vi "Save bline to memory1.vi"(0 "PSOCTSpectral Bline":u16[](array[numeric]), 1 "action":T1=enum."Save(ThorOCT)", 5 "index (row)":i32, 9 "PSOCT Spatial Bline":sgl[](array[numeric]), 11 "error in":errorcluster) -> (15 "error out":errorcluster)   [LabVIEW 2018]
uses:
  Controls/Save Bline to Mem Control.ctl
  Controls/FGV Actions.ctl
  Controls/Queue Manager Actions.ctl
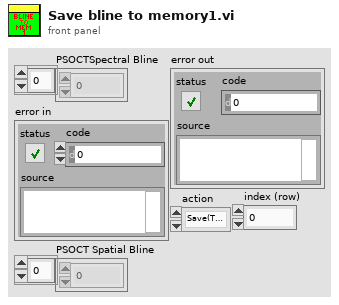
[diagram p1: front panel]
types:
  T1 = typedef "Save Bline to Mem Control.ctl" = enum16{"Output data", "Save(ThorOCT)", "Save(PSOCT)", "FFT and Save", "Uninit", "PSOCT Spectral buffer Set", "PSOCT Spatial buffer Set", "PSOCT Spectral buffer Init", "PSOCT Spatial buffer Init", "ThorOCT Spectral buffer Init", "ThorOCT Spatial buffer Init", "ThorOCT Spectral buffer Set", "ThorOCT Spatial buffer Set", "ThorOCT Spectral Save", "Alazar Spectral Save", "PSOCT save all", "Average"}
  T2 = typedef "FGV Actions.ctl" = enum16{"Init", "Set", "Get", "Clear"}
  T3 = typedef "System Parameters.ctl" = cluster{"Optical Parameters":T4, "Vibratome":T5, "Table Stages":T6, "Imaging Parameter":T9, "Galvo HW Parameters":cluster{"Analog Out Channel":tag, "Min Voltage":dbl, "Max Voltage":dbl, "Pixel Clock Source":tag, "Sample Rate":dbl, "Line Clock Out Ch":tag, "2P ready check":tag}, "Alazar parameters":T11, "Mosaic Paramter":T18, "Manual Controls":T19, "Z stage setting":T23, "Attenuator":T24}
  T4 = typedef "Optical Parameters.ctl" = cluster{"Obj. Focal Length [mm]":dbl, "Scan Lens EFL[mm]":dbl, "Tube Lens EFL[mm]":dbl, "Galvo V Range (+/-)":dbl, "Galvo Max Half Angle [Deg]":dbl, "Max Galvo Range[%]":dbl}
  T5 = typedef "Vibratome Parameters.ctl" = cluster{"Pre Cut Dwell [s]":dbl, "Blade Frequency [RPM]":u16, "Slice Speed [mm/s]":dbl, "Post Cut Dwell [s]":dbl, "Ramp Time [s]":dbl, "Start X [mm]":dbl, "Start Y [mm]":dbl, "Slice Length [mm]":dbl, "Slice Axis":enum16{"X Axis", "Y Axis", "Z Axis"}, "Controller VISA Ref":refnum<visa-resource-name>}
  T6 = typedef "Translation Stage Parameters.ctl" = cluster{"X Stage":T7, "Y Stage":T7, "Z Stage":T7, "Attenuator":T7}
  T7 = typedef "Translation Stage Cluster.ctl" = cluster{"Position":dbl, "Is.Enabled?":bool, "Is.Connected?":bool, "Device SN":string, "AccelerationMaximum":dbl, "VelocityMaximum":dbl, "Acceleration":dbl, "Velocity":dbl, "waitTimeout (ms)":i32, "Model":T8, "Is.Homed?":bool, "MOVE":bool}
  T8 = typedef "Translation Stage Types.ctl" = enum16{"None", "Thorlabs LTS", "Thorlabs MLJ"}
  T9 = typedef "Imaging Parameters.ctl" = cluster{"Raster Scan Direction":T10, "Pixel Dwell Time [Clock Cycles]":u16, "Flyback Time [Clock Cycles]":u16, "XY Center [um]":cluster{"X":dbl, "Y":dbl}, "Pixel Step Size [um] X":dbl, "XY Image Size":enum16{"32 x 32", "64 x 64", "128 x 128", "256 x 256", "512 x 512", "1024 x 1024", "2048 x 2048"}, "Custom":bool, "Custom Size":cluster{"X":u16, "Y":u16}, "Line Averages":u16, "Pixel Step Size [um] Y":dbl}
  T10 = typedef "Scan Direction.ctl" = enum16{"Uni Directional", "Bi Directional", "None"}
  T11 = typedef "Alazar parameters.ctl" = cluster{"Trigger Settings":cluster{"General Trigger Settings":T12, "Trigger Engine 1":T13, "Trigger Engine 2":T13}, "Device ID":T14, "Ch A Input Control":T15, "Ch B Input Control":T15, "Acq Settings":T16, "Capture Clock":T17}
  T12 = typedef "General Trigger Settings.ctl" = cluster{"Trigger Operation":u32, "Coupling ID":u32, "Range ID":u32, "Delay":u32, "Timeout Ticks":u32, "Mode":u32, "Parameter":u32}
  T13 = typedef "Trigger Engine Controls.ctl" = cluster{"Trigger Engine":u32, "Source":u32, "Slope":u32, "Level":u32}
  T14 = typedef "Alazar Device ID.ctl" = cluster{"System ID":u32, "Board ID":u32}
  T15 = typedef "Channel Input Controls.ctl" = cluster{"Channel":u8, "Coupling":u32, "Range":u32, "Impedance":u32}
  T16 = typedef "Alazar Acquisition Settings.ctl" = cluster{"Record Length":u32, "Offset":u32, "Records Per Buffer":u32, "Records Count (Records/Acq)":u32, "Window Type":u32, "Footer":u32, "Samples per record":u32, "Output Format":u32}
  T17 = typedef "Clock Controls.ctl" = cluster{"Sample Rate":u32, "Decimation":u32, "Source":u32, "Edge":u32}
  T18 = typedef "Mosaic Parameter.ctl" = cluster{"X Axis":cluster{"Start [mm]":dbl, "Steps [pts]":dbl, "End [mm]":dbl}, "Y Axis":cluster{"Start [mm]":dbl, "Steps [pts]":dbl, "End [mm]":dbl}, "Scan Pattern":enum16{"Uni-directional", "Bi-Directional", "Spiral Out", "Spiral In"}, "Overlap Options":cluster{"Overlap Type":enum16{"No Overlap", "X Only", "Y Only", "X and Y"}, "Percent Overlap":u8, "Justify":enum16{"Start", "Center", "End"}}}
  T19 = typedef "Manual Controls.ctl" = cluster{"Data Path":path, "Save parameters":T20, "Acquisition mode":T21, "PSOCT Channel":u32, "Save data?":bool, "AIP rotation angle":dbl, "Pause acquisition?":bool, "Outgoing Mail Server (SMTP)":string, "Email":string, "Password":string, "Carrier 1":enum16{"T-Mobile", "AT&T", "Verizon", "Sprint"}, "phone number 1":string, "Subject":string, "Message":string, "Carrier 2":enum16{"T-Mobile", "AT&T", "Verizon", "Sprint"}, "phone number 2":string, "Outputs for GPU FFT":T22, "Slice# init":i32}
  T20 = typedef "FFT parameters.ctl" = cluster{"start pixel":i32, "#pixels to save":i32}
  T21 = typedef "FFT mode.ctl" = enum16{"ThorOCT B line", "ThorOCT Spectral", "ThorOCT FFT", "Alazar B line", "Alazar FFT", "GPU FFT", "Alazar Spectral", "Simulation", "auto adjust focus", "Save all"}
  T22 = typedef "GPU FFT outputs.ctl" = enum16{"Amp + Phase diff", "Amp + Phase", "Amp only"}
  T23 = typedef "Vibratome Param.ctl" = cluster{"first cut height(mm)":dbl, "cut thickness[um]":u32[], "#cycles":u16, "PSOCT thickness(um)":u32[], "First image height(mm)":dbl, "Pause?":bool[], "Z0":dbl, "fixed Z0?":bool, "Cut_aft_2P?(leave empty if no 2P)":bool[], "2P thickness(um) (leave empty if not used)":u32[], "2P_cover_all_depth? (leave empty if no 2P)":bool[]}
  T24 = typedef "attenuator.ctl" = cluster{"Power after Objective (recalibrate every 6 month)":dbl[]}
  T25 = typedef "Queue Manager Actions.ctl" = enum16{"Init", "Enqueue", "Enqueue All", "Preview Queue", "Dequeue", "Get Status", "Flush Queue", "Flush All Queues", "Release All Queues", "Release Queue", "Enqueue at Opposite End"}
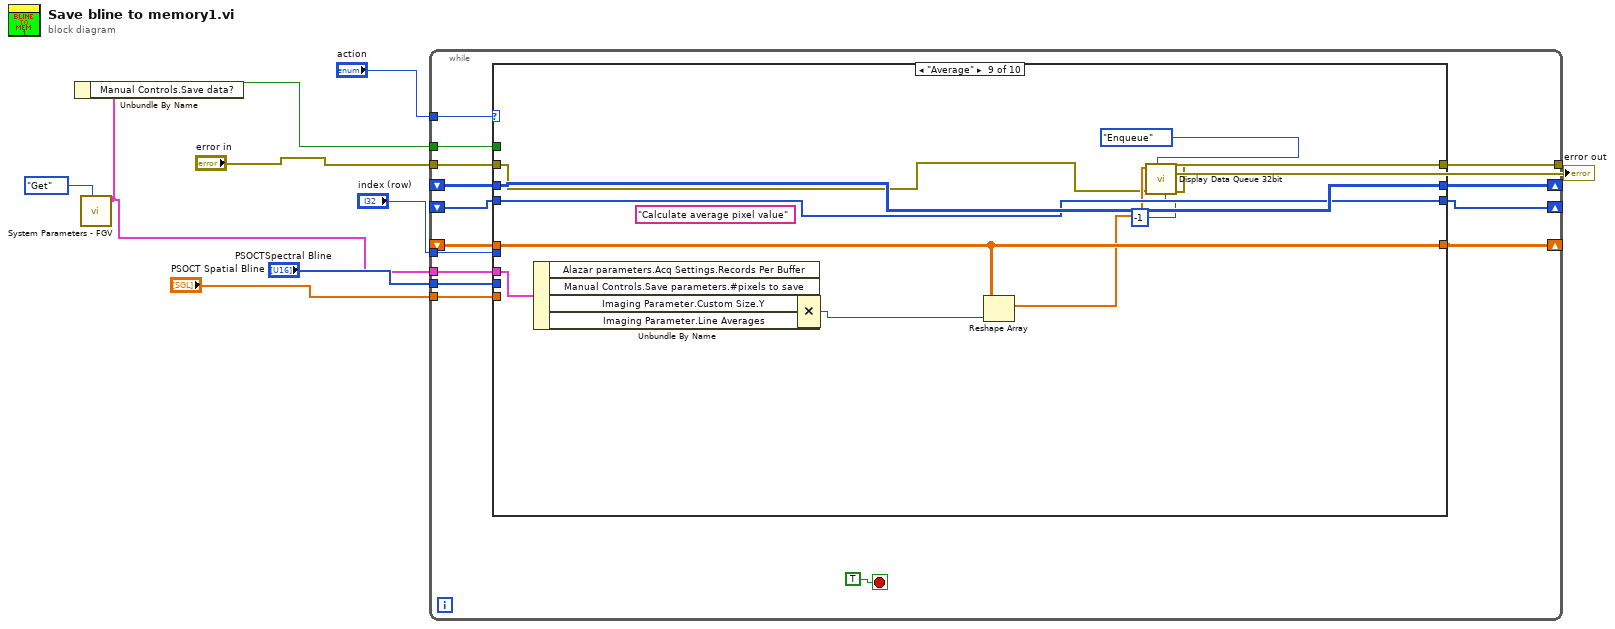
[diagram p0: block diagram]
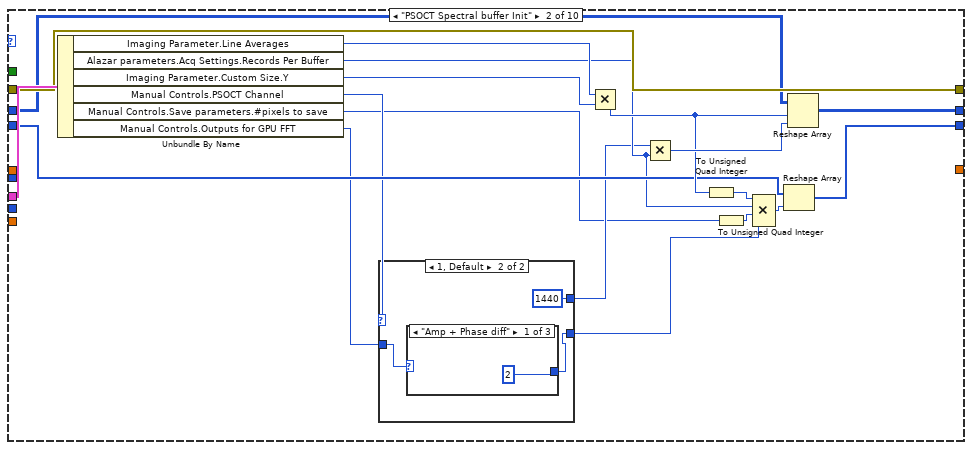
[diagram p3: hidden frame]
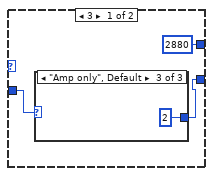
[diagram p4: hidden frame]
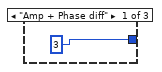
[diagram p5: hidden frame]
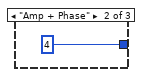
[diagram p6: hidden frame]
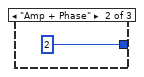
[diagram p7: hidden frame]
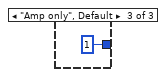
[diagram p8: hidden frame]
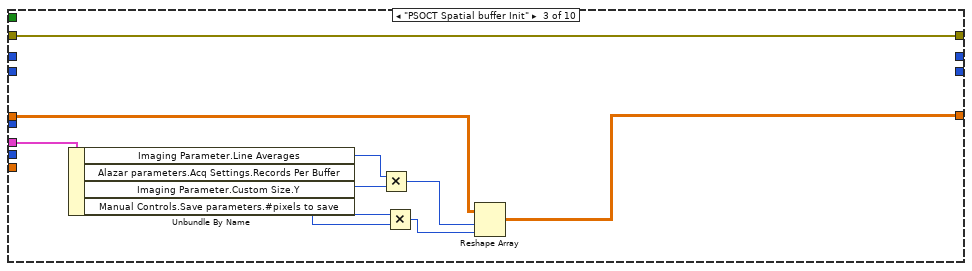
[diagram p9: hidden frame]
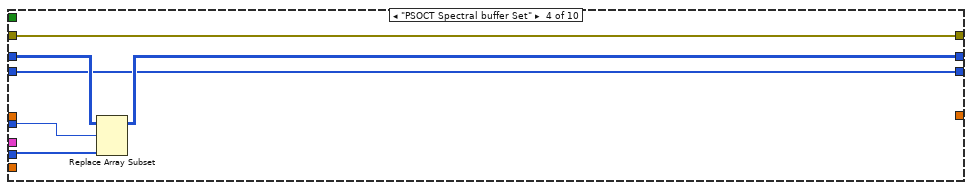
[diagram p10: hidden frame]
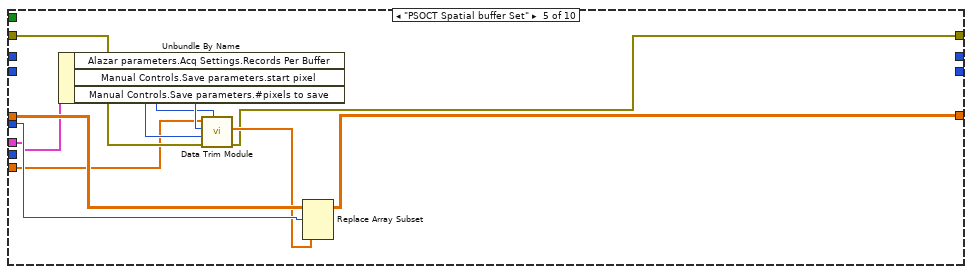
[diagram p11: hidden frame]
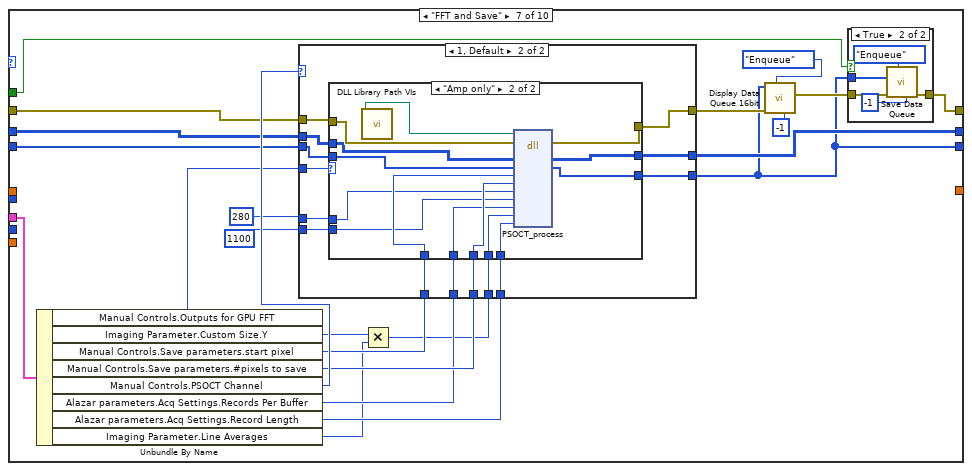
[diagram p13: hidden frame]
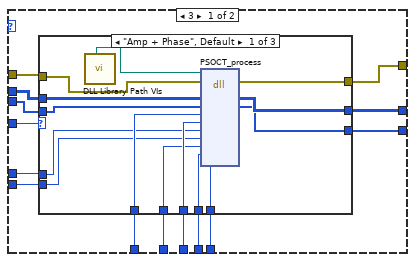
[diagram p14: hidden frame]
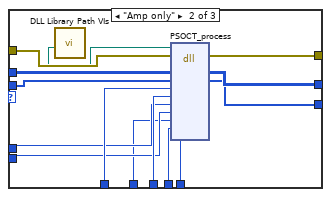
[diagram p15: hidden frame]
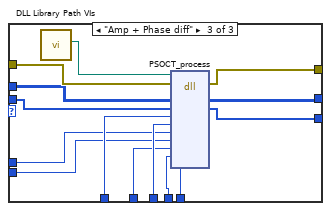
[diagram p16: hidden frame]
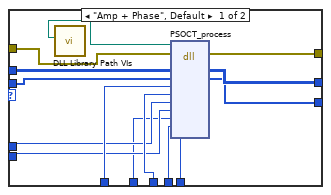
[diagram p17: hidden frame]
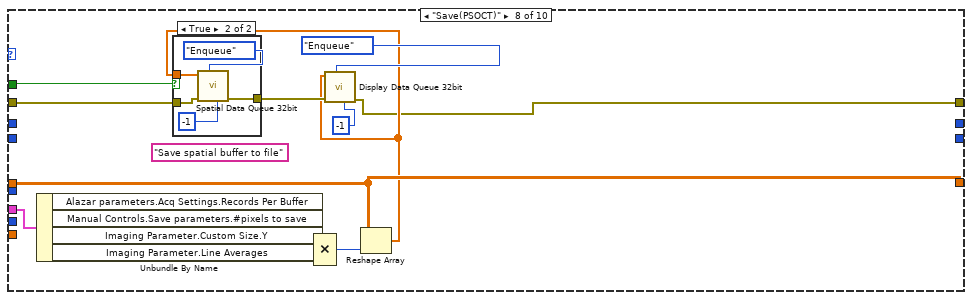
[diagram p19: hidden frame]
diagram:
  n1 = call "System Parameters - FGV.vi"("Actions"=FGV_Actions."Get") -> ("System Parameters [Out]"=w2:T3)  [unwired: 9 in, 1 out]
  n2 = Unbundle By Name(w2) -> ("Manual Controls.Save data?"=w1:bool)
  n3 = while {
    tunnel: "action" -> [w10]
    shift-right: [w22] -> _
    shift-left: _ -> [w17]
    tunnel: "PSOCTSpectral Bline" -> [w13]
    tunnel: "index (row)" -> [w11]
    tunnel: "error in" -> [w16]
    tunnel: w2 -> [w12]
    tunnel: [w23] -> w4
    shift-right: [w20] -> _
    shift-left: _ -> [w19]
    tunnel: "PSOCT Spatial Bline" -> [w14]
    tunnel: w1 -> [w15]
    shift-right: [w21] -> _
    shift-left: _ -> [w18]
    stop <- TRUE stop-if-true
    n4 = case shown="\"Average\"" w10 {
      tunnel: [w28 w46 _ w72 _ _ w96 _ w240 w248] -> w22
      tunnel: w17 -> [w28 w37 _ w75 _ _ w105 _ w240 w248]
      tunnel: w13 -> [_ _ _ w73 _ _ _ _ _ _]
      tunnel: w11 -> [_ _ _ w74 w84 _ _ _ _ _]
      tunnel: w16 -> [w26 w42 w64 w71 w80 w87 w106 w227 w234 w251]
      tunnel: w12 -> [_ w45 w69 _ w81 _ w109 w225 w246 _]
      tunnel: [w26 w42 w64 w71 w76 w87 w95 w214 w235 w250] -> w23
      tunnel: [w27 _ w63 _ w85 _ _ w226 w247 _] -> w20
      tunnel: w19 -> [w27 _ w62 _ w86 _ _ w226 w247 _]
      tunnel: w14 -> [_ _ _ _ w78 _ _ _ _ _]
      tunnel: w15 -> [_ _ _ _ _ _ w108 w217 _ _]
      tunnel: [w25 w41 _ w70 _ _ w91 _ w239 _] -> w21
      tunnel: w18 -> [w25 w36 _ w70 _ _ w104 _ w239 _]
      frame Default {
      }
      frame "PSOCT Spectral buffer Init" {
        n5 = Unbundle By Name(w45) -> ("Imaging Parameter.Line Averages"=w44:u16, "Alazar parameters.Acq Settings.Records Per Buffer"=w34:u32, "Imaging Parameter.Custom Size.Y"=w43:u16, "Manual Controls.PSOCT Channel"=w31:u32, "Manual Controls.Save parameters.#pixels to save"=w30:i32, "Manual Controls.Outputs for GPU FFT"=w29:T22)
        n6 = case shown="1, Default" w31 {
          tunnel: [w50 w56] -> w38
          tunnel: w29 -> [w49 w55]
          tunnel: [u32 2880 ("element") u32 1440 ("element")] -> w32
          frame 3 {
            n7 = case shown="\"Amp only\", Default" w49 {
              tunnel: [3 u64 4 ("element") u64 2 ("element")] -> w50
              frame "Amp + Phase diff" {
              }
              frame "Amp + Phase" {
              }
              frame "Amp only", Default {
              }
            }
          }
          frame 1, Default {
            n8 = case shown="\"Amp + Phase diff\"" w55 {
              tunnel: [2 u64 2 ("element") u64 1 ("element")] -> w56
              frame "Amp + Phase diff" {
              }
              frame "Amp + Phase" {
              }
              frame "Amp only", Default {
              }
            }
          }
        }
        n9 = Multiply(x=w44, y=w43) -> (x*y=w40:u16)
        n10 = Multiply(x=w32, y=w34) -> (x*y=w47:u32)
        n11 = To Unsigned Quad Integer(1:w40) -> (0:w35:u64)
        n12 = To Unsigned Quad Integer(1:w30) -> (0:w33:u64)
        n13 = Compound Arithmetic op=MULTIPLY(w35, w34, w33, w38) -> (w39:u64)
        n14 = Reshape Array(w36, w39) -> (w41:u16[])
        n15 = Reshape Array(w37, w40, w47) -> (w46:u16[][])
      }
      frame "PSOCT Spatial buffer Init" {
        n16 = Unbundle By Name(w69) -> ("Imaging Parameter.Line Averages"=w66:u16, "Alazar parameters.Acq Settings.Records Per Buffer"=w67:u32, "Imaging Parameter.Custom Size.Y"=w65:u16, "Manual Controls.Save parameters.#pixels to save"=w68:i32)
        n17 = Multiply(x=w66, y=w65) -> (x*y=w61:u16)
        n18 = Multiply(x=w67, y=w68) -> (x*y=w60:u32)
        n19 = Reshape Array(w62, w61, w60) -> (w63:sgl[][])
      }
      frame "PSOCT Spectral buffer Set" {
        n20 = Replace Array Subset(array=w75, new element=w73, index (row)=w74) -> (w72:u16[][])  [unwired: 1 in]
      }
      frame "PSOCT Spatial buffer Set" {
        n21 = Unbundle By Name(w81) -> ("Alazar parameters.Acq Settings.Records Per Buffer"=w83:u32, "Manual Controls.Save parameters.start pixel"=w82:i32, "Manual Controls.Save parameters.#pixels to save"=w77:i32)
        n22 = call "Data Trim Module.vi"("#pixels to save"=w77, "error in"=w80, "start pixel"=w82, "#A-lines"=w83, "1D Array in"=w78) -> ("error out"=w76:errorcluster, "array for saving"=w79:sgl[])  [unwired: 5 in]
        n23 = Replace Array Subset(array=w86, new element=w79, index (row)=w84) -> (w85:sgl[][])  [unwired: 1 in]
      }
      frame "Uninit" {
      }
      frame "FFT and Save" {
        n24 = Unbundle By Name(w109) -> ("Manual Controls.Outputs for GPU FFT"=w97:T22, "Imaging Parameter.Custom Size.Y"=w90:u16, "Manual Controls.Save parameters.start pixel"=w103:i32, "Manual Controls.Save parameters.#pixels to save"=w102:i32, "Manual Controls.PSOCT Channel"=w107:u32, "Alazar parameters.Acq Settings.Records Per Buffer"=w99:u32, "Alazar parameters.Acq Settings.Record Length"=w98:u32, "Imaging Parameter.Line Averages"=w89:u16)
        n25 = Multiply(x=w90, y=w89) -> (x*y=w88:u16)
        n26 = case shown="1, Default" w107 {
          tunnel: w106 -> [w123 w179]
          tunnel: w105 -> [w122 w178]
          tunnel: w104 -> [w121 w177]
          tunnel: w103 -> [w120 w176]
          tunnel: w102 -> [w119 w175]
          tunnel: i16 280 ("a") -> [w118 w174]
          tunnel: i16 1100 ("b") -> [w117 w173]
          tunnel: w99 -> [w116 w172]
          tunnel: w88 -> [w115 w171]
          tunnel: w98 -> [w114 w170]
          tunnel: [w111 w167] -> w93
          tunnel: [w110 w166] -> w96
          tunnel: [w113 w169] -> w91
          tunnel: w97 -> [w112 w168]
          frame 3 {
            n27 = case shown="\"Amp + Phase\", Default" w112 {
              tunnel: w123 -> [w137 w151 w165]
              tunnel: w122 -> [w134 w148 w164]
              tunnel: w121 -> [w133 w147 w163]
              tunnel: w120 -> [w132 w146 w162]
              tunnel: w119 -> [w131 w145 w161]
              tunnel: w118 -> [w130 w144 w160]
              tunnel: w117 -> [w129 w143 w159]
              tunnel: w116 -> [w128 w142 w158]
              tunnel: w115 -> [w127 w141 w157]
              tunnel: w114 -> [w126 w140 w156]
              tunnel: [w125 w139 w155] -> w111
              tunnel: [w136 w150 w154] -> w110
              tunnel: [w135 w149 w153] -> w113
              frame "Amp + Phase", Default {
                n28 = call "DLL Library Path VIs.vi"() -> ("GPU FFT amp amp phase phase"=w124:path)  [unwired: 5 in, 6 out]
                n29 = dll-call lib="C:/Project/SerialSectionOCT/SerialSectOCT/Labview Software/DLL/CUDA_FFT_2_channel_amp_amp_phase_phase.dll" fn="PSOCT_process"(path in=w124, error in=w137, "h_signal"=w134, "h_processed_signal"=w133, "Z0"=w132, "DEPTH"=w131, "a"=w130, "b"=w129, "NALINES"=w128, "NBLINES"=w127, "SAMPLES"=w126) -> (error out=w125:errorcluster, "h_signal"=w136:u16[][], "h_processed_signal"=w135:u16[])  [unwired: 9 in, 1 out]
              }
              frame "Amp only" {
                n30 = call "DLL Library Path VIs.vi"() -> ("GPU FFT amp amp"=w138:path)  [unwired: 5 in, 6 out]
                n31 = dll-call lib="C:/Project/SerialSectionOCT/SerialSectOCT/Labview Software/DLL/CUDA_FFT_2_channel_amp_amp.dll" fn="PSOCT_process"(path in=w138, error in=w151, "h_signal"=w148, "h_processed_signal"=w147, "Z0"=w146, "DEPTH"=w145, "a"=w144, "b"=w143, "NALINES"=w142, "NBLINES"=w141, "SAMPLES"=w140) -> (error out=w139:errorcluster, "h_signal"=w150:u16[][], "h_processed_signal"=w149:u16[])  [unwired: 9 in, 1 out]
              }
              frame "Amp + Phase diff" {
                n32 = call "DLL Library Path VIs.vi"() -> ("GPU FFT amp amp phase diff"=w152:path)  [unwired: 5 in, 6 out]
                n33 = dll-call lib="C:/Project/SerialSectionOCT/SerialSectOCT/Labview Software/DLL/CUDA_FFT_2_channel_amp_amp_phasediff.dll" fn="PSOCT_process"(path in=w152, error in=w165, "h_signal"=w164, "h_processed_signal"=w163, "Z0"=w162, "DEPTH"=w161, "a"=w160, "b"=w159, "NALINES"=w158, "NBLINES"=w157, "SAMPLES"=w156) -> (error out=w155:errorcluster, "h_signal"=w154:u16[][], "h_processed_signal"=w153:u16[])  [unwired: 9 in, 1 out]
              }
            }
          }
          frame 1, Default {
            n34 = case shown="\"Amp only\"" w168 {
              tunnel: w179 -> [w193 w207]
              tunnel: w178 -> [w190 w206]
              tunnel: w177 -> [w189 w205]
              tunnel: w176 -> [w188 w204]
              tunnel: w175 -> [w187 w203]
              tunnel: w174 -> [w186 w202]
              tunnel: w173 -> [w185 w201]
              tunnel: w172 -> [w184 w200]
              tunnel: w171 -> [w183 w199]
              tunnel: w170 -> [w182 w198]
              tunnel: [w181 w197] -> w167
              tunnel: [w192 w196] -> w166
              tunnel: [w191 w195] -> w169
              frame "Amp + Phase", Default {
                n35 = call "DLL Library Path VIs.vi"() -> ("GPU FFT single amp phase"=w180:path)  [unwired: 5 in, 6 out]
                n36 = dll-call lib="C:/Project/SerialSectionOCT/SerialSectOCT/Labview Software/DLL/CUDA_FFT_1_channel_amp_phase.dll" fn="PSOCT_process"(path in=w180, error in=w193, "h_signal"=w190, "h_processed_signal"=w189, "Z0"=w188, "DEPTH"=w187, "a"=w186, "b"=w185, "NALINES"=w184, "NBLINES"=w183, "SAMPLES"=w182) -> (error out=w181:errorcluster, "h_signal"=w192:u16[][], "h_processed_signal"=w191:u16[])  [unwired: 9 in, 1 out]
              }
              frame "Amp only" {
                n37 = call "DLL Library Path VIs.vi"() -> ("GPU FFT single amp"=w194:path)  [unwired: 5 in, 6 out]
                n38 = dll-call lib="C:/Project/SerialSectionOCT/SerialSectOCT/Labview Software/DLL/CUDA_FFT_1_channel_amp.dll" fn="PSOCT_process"(path in=w194, error in=w207, "h_signal"=w206, "h_processed_amps"=w205, "Z0"=w204, "DEPTH"=w203, "a"=w202, "b"=w201, "NALINES"=w200, "NBLINES"=w199, "SAMPLES"=w198) -> (error out=w197:errorcluster, "h_signal"=w196:u16[][], "h_processed_amps"=w195:u16[])  [unwired: 9 in, 1 out]
              }
            }
          }
        }
        n39 = call "Display Data Queue 16bit.vi"("timeout in ms (-1)"=-1, "Action"=Queue_Manager_Actions."Enqueue", "data in"=w91) -> ()  [unwired: 5 in, 4 out]
        n40 = case shown="True" w108 {
          tunnel: w93 -> [w208 w213]
          tunnel: [w208 w212] -> w95
          tunnel: w91 -> [_ w209]
          frame False {
          }
          frame True {
            n41 = call "Save Data Queue.vi"("timeout in ms (-1)"=-1, "Action"=Queue_Manager_Actions."Enqueue", "error in (no error)"=w213, "data in"=w209) -> ("error out"=w212:errorcluster)  [unwired: 4 in, 3 out]
          }
        }
      }
      frame "Save(PSOCT)" {
        (unwired) "Save spatial buffer to file"
        n42 = Unbundle By Name(w225) -> ("Alazar parameters.Acq Settings.Records Per Buffer"=w224:u32, "Manual Controls.Save parameters.#pixels to save"=w223:i32, "Imaging Parameter.Custom Size.Y"=w222:u16, "Imaging Parameter.Line Averages"=w216:u16)
        n43 = Compound Arithmetic op=MULTIPLY(w224, w223, w222, w216) -> (w221:u32)
        n44 = Reshape Array(w226, w221) -> (w215:sgl[])
        n45 = case shown="True" w217 {
          tunnel: w227 -> [w228 w233]
          tunnel: [w228 w232] -> w220
          tunnel: w215 -> [_ w229]
          frame False {
          }
          frame True {
            n46 = call "Spatial Data Queue 32bit.vi"("timeout in ms (-1)"=-1, "Action"=Queue_Manager_Actions."Enqueue", "error in (no error)"=w233, "data in"=w229) -> ("error out"=w232:errorcluster)  [unwired: 4 in, 3 out]
          }
        }
        n47 = call "Display Data Queue 32bit.vi"("timeout in ms (-1)"=-1, "Action"=Queue_Manager_Actions."Enqueue", "error in (no error)"=w220, "data in"=w215) -> ("error out"=w214:errorcluster)  [unwired: 4 in, 3 out]
      }
      frame "Average" {
        (unwired) "Calculate average pixel value"
        n48 = Unbundle By Name(w246) -> ("Alazar parameters.Acq Settings.Records Per Buffer"=w245:u32, "Manual Controls.Save parameters.#pixels to save"=w244:i32, "Imaging Parameter.Custom Size.Y"=w243:u16, "Imaging Parameter.Line Averages"=w241:u16)
        n49 = Compound Arithmetic op=MULTIPLY(w245, w244, w243, w241) -> (w242:u32)
        n50 = Reshape Array(w247, w242) -> (w236:sgl[])
        n51 = call "Display Data Queue 32bit.vi"("timeout in ms (-1)"=-1, "Action"=Queue_Manager_Actions."Enqueue", "error in (no error)"=w234, "data in"=w236) -> ("error out"=w235:errorcluster)  [unwired: 4 in, 3 out]
      }
      frame "Alazar Spectral Save" {
        n52 = call "Spectral Save Queue.vi"("timeout in ms (-1)"=-1, "Action"=Queue_Manager_Actions."Enqueue", "error in (no error)"=w251, "data in"=w248) -> ("error out"=w250:errorcluster)  [unwired: 4 in, 3 out]
      }
    }
  }
  "error out" <- w4
